vi "Read Attributes.vi"(11 "Return VF Setpoint Msg":refnum<class "Return VF Setpoint Msg.lvclass">) -> (2 "Payload":T1)   [LabVIEW 2016, in "Optimization Framework.lvlib" / "Return VF Setpoint Msg.lvclass"]
uses:
  Return VF Setpoint Msg.lvclass
  Return VF Setpoint Msg.lvclass/Return VF Setpoint Msg.ctl
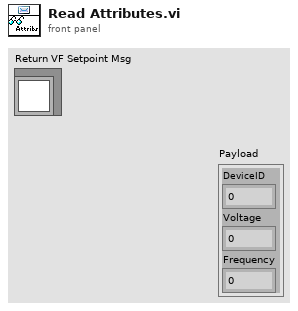
[diagram p1: front panel]
types:
  T1 = cluster{"DeviceID":u64, "Voltage":dbl, "Frequency":dbl}
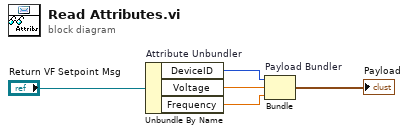
[diagram p0: block diagram]
diagram:
  n1 = Unbundle By Name "Attribute Unbundler"("Return VF Setpoint Msg") -> ("DeviceID"=w1:u64, "Voltage"=w3:dbl, "Frequency"=w2:dbl)
  n2 = Bundle "Payload Bundler"("DeviceID"=w1, "Voltage"=w3, "Frequency"=w2) -> (→"Payload":T1)  [unwired: 1 in]
